vi "sub_prepare_HexPlot_command.vi"(10 "Dynamic data":T1, 11 "Input parameters":T2={"Measurement type"=enum."Debug", "Sensor type"=enum."HPK_8in_271ch", "Identifier"="test.txt", "Open after execution?"=FALSE, "Plot after execution?"=FALSE, "Display channel"=0, "Voltage Delay (s)"=0.5, "Switch Delay (s)"=0.01, "VISA resource name source"="", "VISA resource name DMM"="", "VISA resource name LCR"="", "Compliance  Level (A)"=10.0, "Voltage Limit (V)"=1000.0, "Data storage location"="", "Scan voltages"="", "Use source as DMM?"=FALSE, "LCR signal frequenzy (Hz)"=10.0, "DMM device"=enum."Keithley2001", "Sampling number"=1, "Use env. sensors on"=enum."Sensirion sht1x/7x", "Switchboard Handle"=0, "Use Switchboard"=FALSE, "LCR signal voltage (V)"=10000.0, "Repeat"=1, "Scan voltages IV"="", "Scan voltages CV"="", "Hex pad numbers?"=FALSE, "Set measurement type"=enum."Debug", "Custom pad scan"="", "IV voltage Delay (s)"=0.5, "CV voltage Delay (s)"=0.5, "Needle measurement?"=FALSE, "Comments"="test.txt", "LCR signal frequenzy (kHz)"=10.0, "Compliance  Level (uA)"=10.0, "Open Correction Array"=array2304x3[6912 elements], "Current set voltage"=0.0, "Last set voltage"=0.0, "Current channel"=0, "Last OpenCorrection index"=-1, "Total curr/vltg every x steps"=10, "Current channel iteration"=0, "No CV corrections"=FALSE, "Mapfile"="", "Corrfile"="", "IV voltage file"=path "", "CV voltage file"=path "", "IV Switch Delay (s)"=0.01, "CV Switch Delay (s)"=0.01, "Invert polarity"=FALSE, "Set debug dirs"=FALSE, "Is n on p"=FALSE, "Source interlock?"=TRUE, "Voltage file used?"=FALSE, "Pad mask"="", "Mask pad above (uA)"=1.0, "LCR device"=enum."LCR_E4980", "Source device"=enum."Source_2410", "HexPlot binary path"="", "PadReductionFactor"=1.0, "Temperature degC"="", "Fluence [neq]"="", "Annealing [min]"=""} {"CV Switch Delay (s)" format="%#_13g"; "IV Switch Delay (s)" format="%#_13g"; "Last set voltage" format="%#_13g"; "Current set voltage" format="%#_13g"; "CV voltage Delay (s)" format="%#_13g"; "IV voltage Delay (s)" format="%#_13g"; "Voltage Limit (V)" format="%#_13g"; "Voltage Delay (s)" format="%#_13g"; "Switch Delay (s)" format="%#_13g"}) -> (2 "Dynamic data out":T1)   [LabVIEW 2020]
doc: "Set HexPlot command for data display."
uses:
  input_params.ctl
  data_dynamic.ctl
panel:
  out "HexPlot analysis command":string
  out "HexPlot matrix command":string
  out "HexPlot command":string
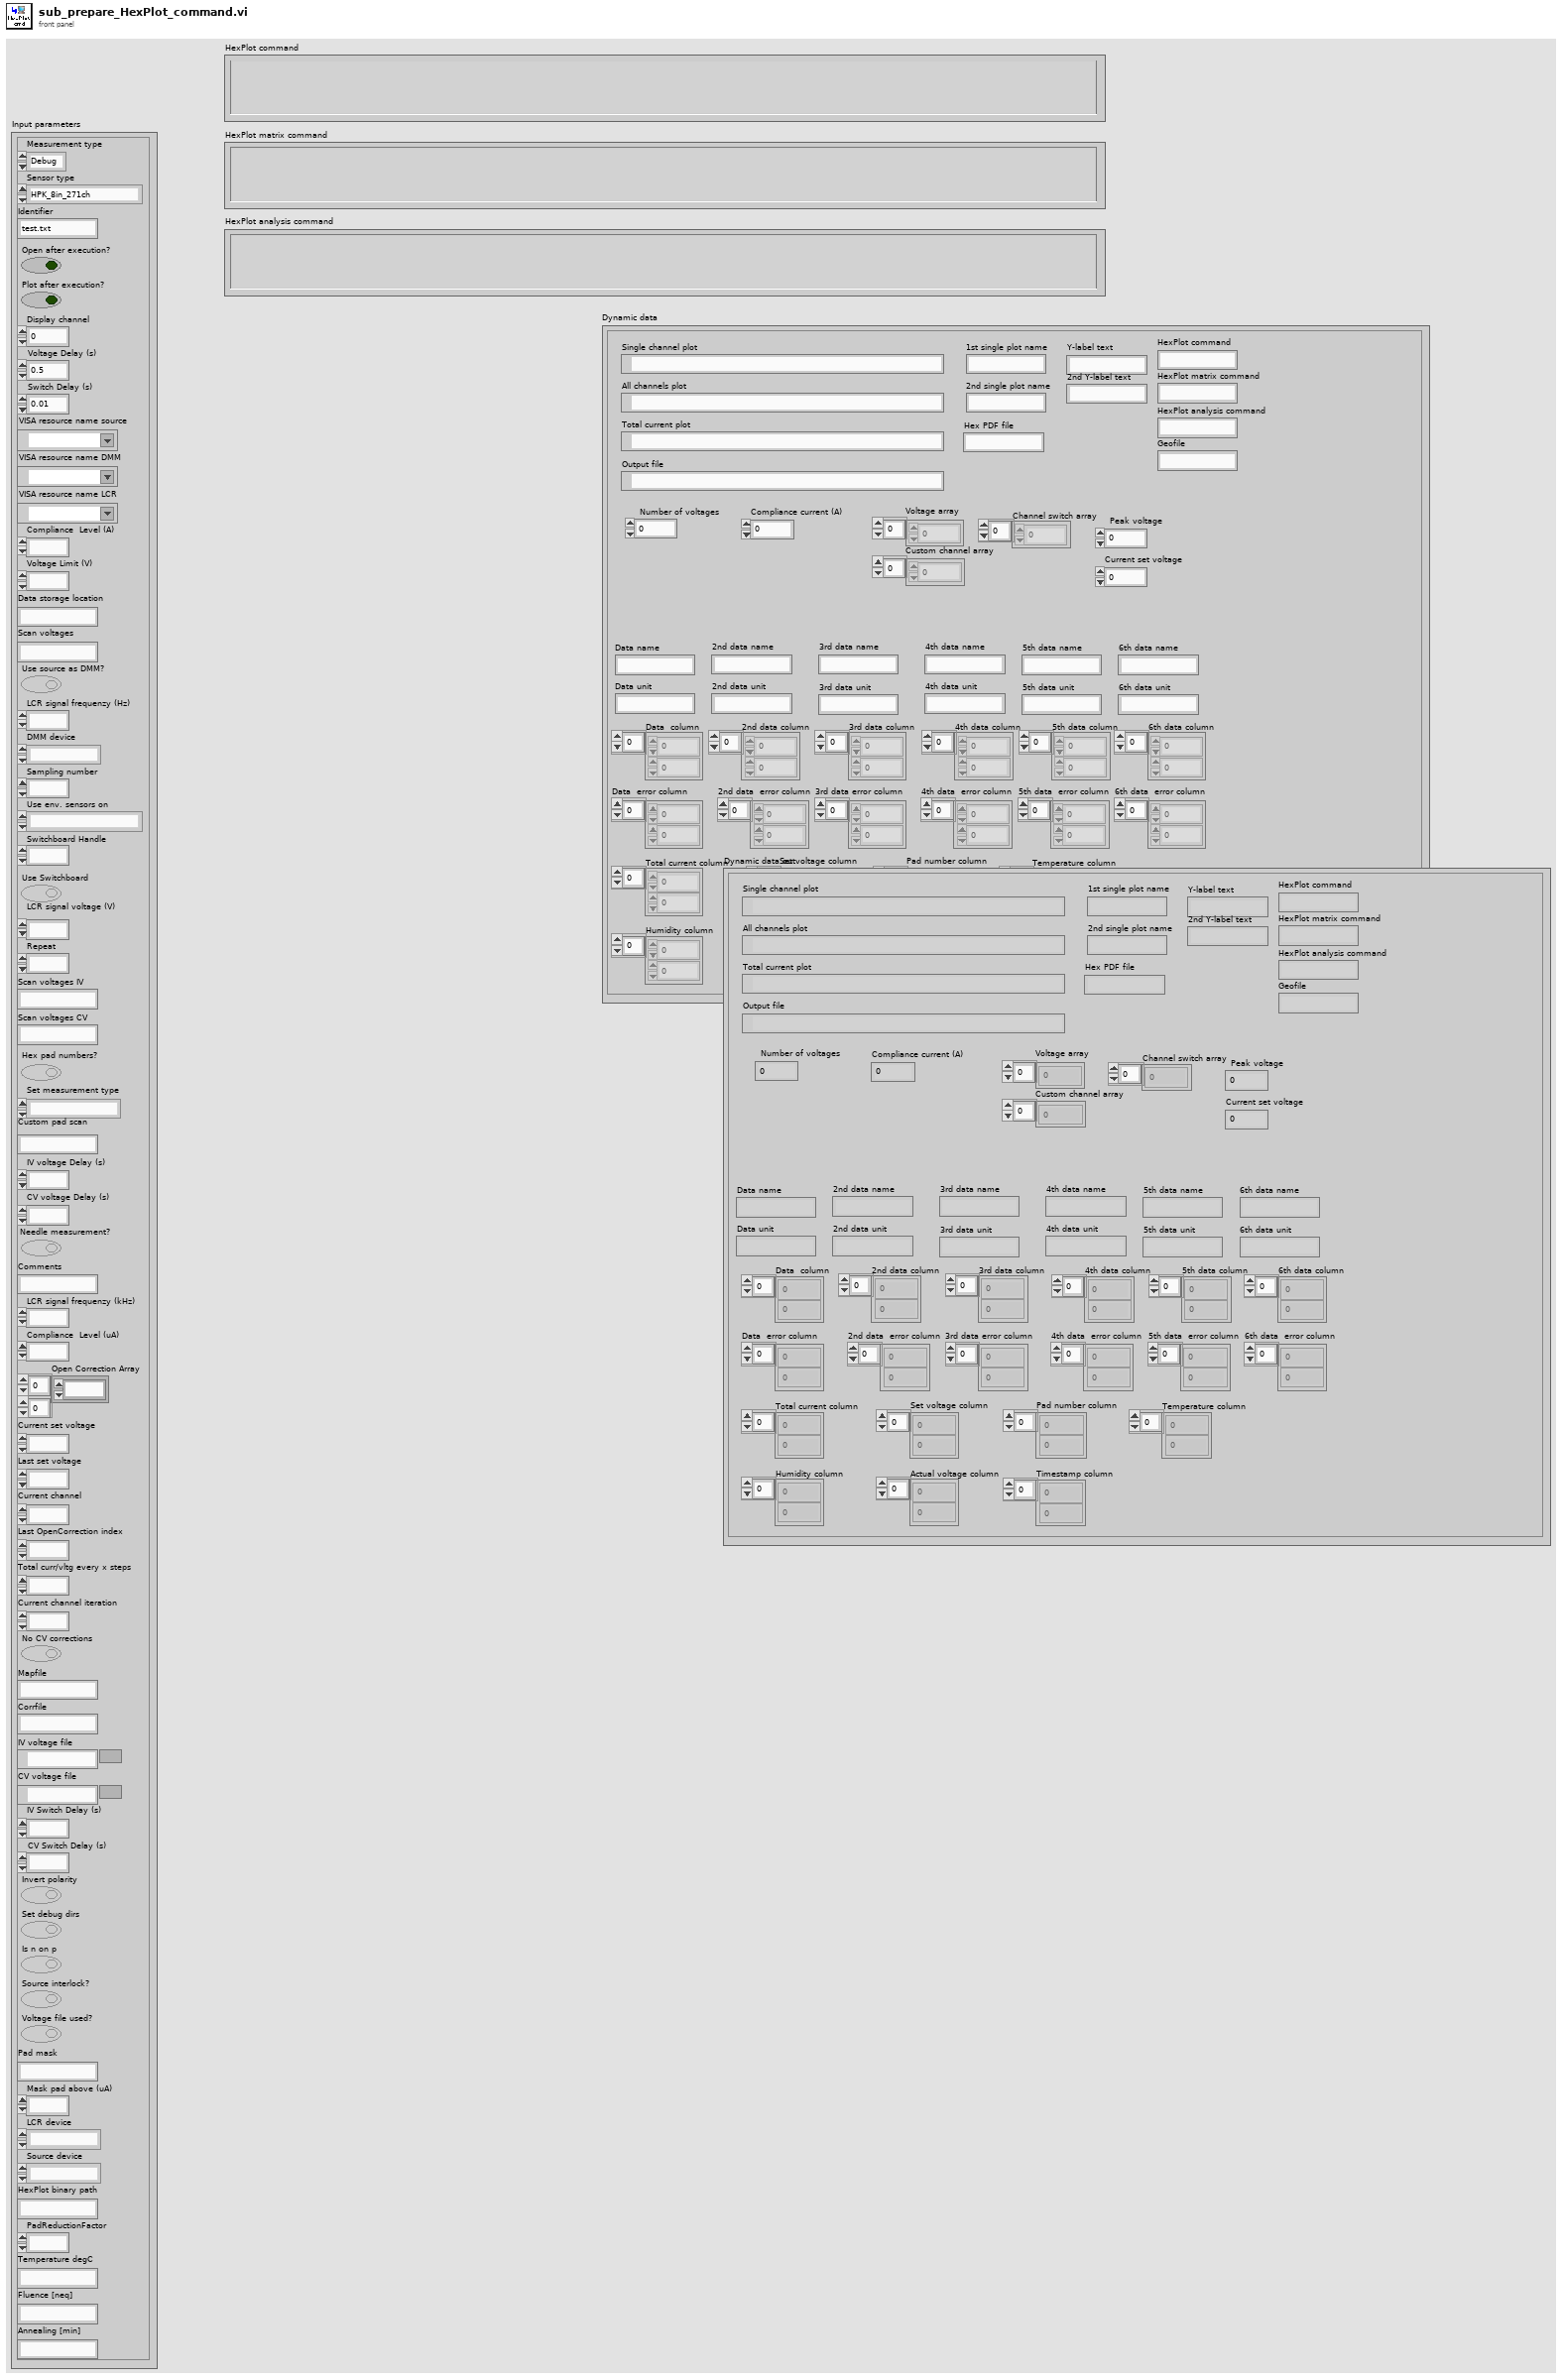
[diagram p1: front panel]
types:
  T1 = typedef "data_dynamic.ctl" = cluster{"Output file":path, "Y-label text":string, "Current set voltage":dbl, "Set voltage column":dbl[], "Pad number column":dbl[], "Data  column":dbl[], "Number of voltages":i32, "Compliance current (A)":dbl, "Geofile":string, "Peak voltage":dbl, "Hex PDF file":string, "Voltage array":dbl[], "Total current column":dbl[], "Timestamp column":dbl[], "Data name":string, "Data unit":string, "2nd data column":dbl[], "2nd data name":string, "2nd data unit":string, "3rd data column":dbl[], "4th data column":dbl[], "3rd data name":string, "3rd data unit":string, "4th data name":string, "4th data unit":string, "Actual voltage column":dbl[], "2nd Y-label text":string, "Single channel plot":path, "Temperature column":dbl[], "Humidity column":dbl[], "Channel switch array":i32[], "1st single plot name":string, "2nd single plot name":string, "All channels plot":path, "HexPlot command":string, "Custom channel array":i32[], "Data  error column":dbl[], "2nd data  error column":dbl[], "3rd data error column":dbl[], "4th data  error column":dbl[], "Total current plot":path, "5th data column":dbl[], "5th data  error column":dbl[], "6th data column":dbl[], "6th data  error column":dbl[], "5th data name":string, "5th data unit":string, "6th data name":string, "6th data unit":string, "HexPlot matrix command":string, "HexPlot analysis command":string}
  T2 = typedef "input_params.ctl" = cluster{"Measurement type":enum16{"IV", "CV", "Debug", "Test_contact"}, "Sensor type":enum16{"HPK_6in_135ch", "HPK_8in_271ch", "IFX_8in_256ch", "Diode", "HPK_6in_239ch", "Full_Matrix", "HPK_8in_271ch_full", "LumiCal", "HPK_8in_444ch", "HPK_8in_198ch_2019", "HPK_8in_MGW_LD_full", "HPK_8in_MGW_LD_a_type_top", "HPK_8in_MGW_LD_a_type_bottom", "HPK_8in_MGW_LD_b_type_left", "HPK_8in_MGW_LD_b_type_right", "HPK_8in_MGW_LD_c_type_left", "HPK_8in_MGW_LD_c_type_right", "HPK_8in_MGW_HD_full", "HPK_8in_MGW_HD_a_type_top", "HPK_8in_MGW_HD_a_type_bottom", "HPK_8in_MGW_HD_b_type_left", "HPK_8in_MGW_HD_b_type_right", "HPK_8in_MGW_HD_c_type_left", "HPK_8in_MGW_HD_c_type_right", "CALICE_6in_256ch"}, "Identifier":string, "Open after execution?":bool, "Plot after execution?":bool, "Display channel":i32, "Voltage Delay (s)":dbl, "Switch Delay (s)":dbl, "VISA resource name source":refnum<visa-resource-name>, "VISA resource name DMM":refnum<visa-resource-name>, "VISA resource name LCR":refnum<visa-resource-name>, "Compliance  Level (A)":dbl, "Voltage Limit (V)":dbl, "Data storage location":string, "Scan voltages":string, "Use source as DMM?":bool, "LCR signal frequenzy (Hz)":dbl, "DMM device":enum16{"Keithley2001", "Keithley2450", "Keithley2410", "Keithley6485", "Keithley6487", "Keithley6517"}, "Sampling number":i32, "Use env. sensors on":enum16{"Sensirion sht1x/7x", "Switch Matrix", "Probecard"}, "Switchboard Handle":u32, "Use Switchboard":bool, "LCR signal voltage (V)":dbl, "Repeat":i32, "Scan voltages IV":string, "Scan voltages CV":string, "Hex pad numbers?":bool, "Set measurement type":enum16{"IV", "CV", "Debug", "Test_contact", "IV+CV"}, "Custom pad scan":string, "IV voltage Delay (s)":dbl, "CV voltage Delay (s)":dbl, "Needle measurement?":bool, "Comments":string, "LCR signal frequenzy (kHz)":dbl, "Compliance  Level (uA)":dbl, "Open Correction Array":dbl[][], "Current set voltage":dbl, "Last set voltage":dbl, "Current channel":i32, "Last OpenCorrection index":i32, "Total curr/vltg every x steps":i32, "Current channel iteration":i32, "No CV corrections":bool, "Mapfile":string, "Corrfile":string, "IV voltage file":path, "CV voltage file":path, "IV Switch Delay (s)":dbl, "CV Switch Delay (s)":dbl, "Invert polarity":bool, "Set debug dirs":bool, "Is n on p":bool, "Source interlock?":bool, "Voltage file used?":bool, "Pad mask":string, "Mask pad above (uA)":dbl, "LCR device":enum16{"LCR_E4980", "AGILENT_4263X"}, "Source device":enum16{"Source_2410", "Source_6487", "Source_2470"}, "HexPlot binary path":string, "PadReductionFactor":dbl, "Temperature degC":string, "Fluence [neq]":string, "Annealing [min]":string}
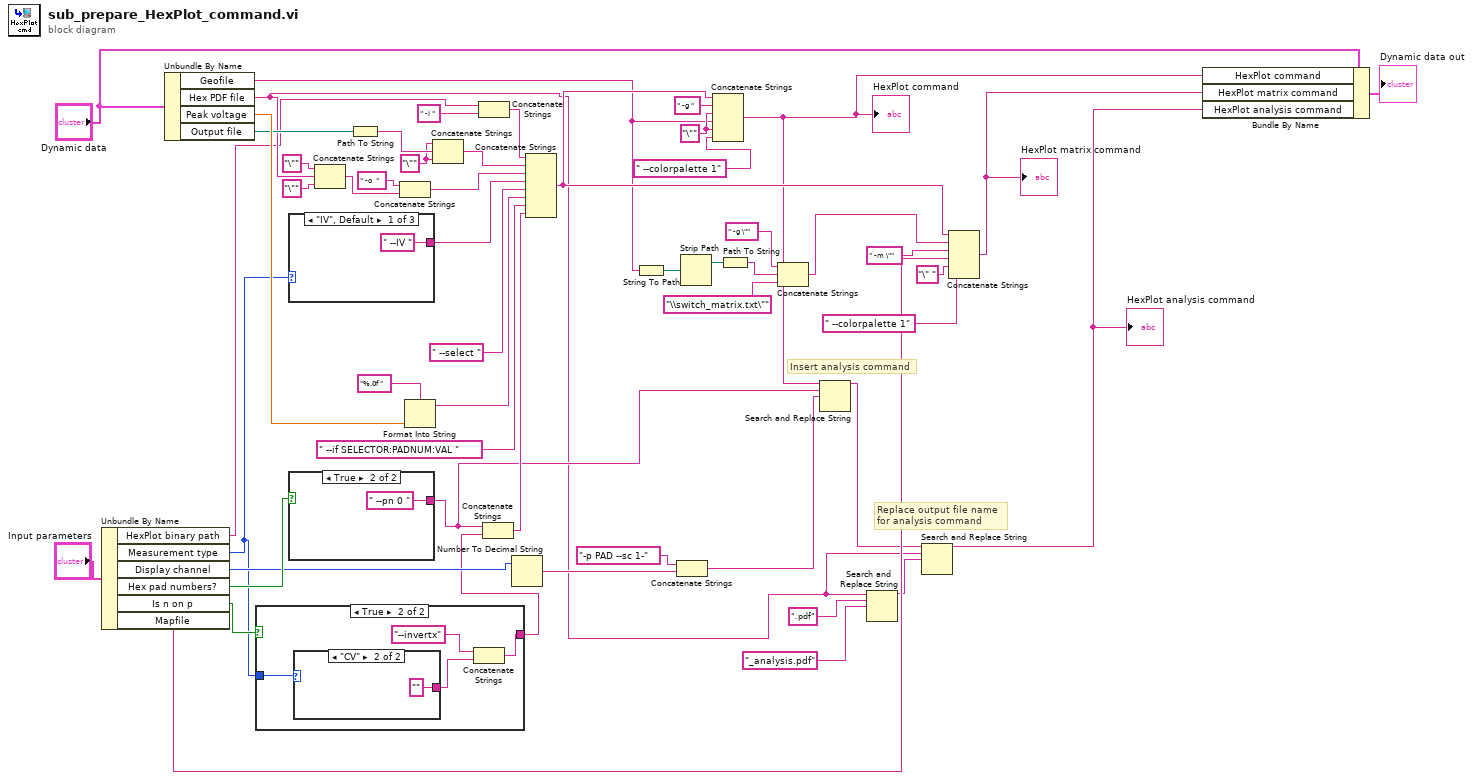
[diagram p0: block diagram]
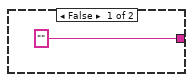
[diagram p2: hidden frame]
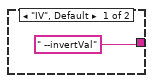
[diagram p3: hidden frame]
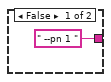
[diagram p4: hidden frame]
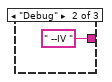
[diagram p5: hidden frame]
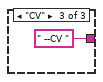
[diagram p6: hidden frame]
diagram:
  w33 = "\"" ("string")
  w32 = "\"" ("string")
  # "Replace output file name\nfor analysis command"
  # "Insert analysis command"
  n1 = Unbundle By Name("Input parameters") -> ("HexPlot binary path"=w3:string, "Measurement type"=w7:enum16{"IV", "CV", "Debug", "Test_contact"}, "Display channel"=w16:i32, "Hex pad numbers?"=w40:bool, "Is n on p"=w21:bool, "Mapfile"=w34:string)
  n2 = Unbundle By Name("Dynamic data") -> ("Geofile"=w29:string, "Hex PDF file"=w9:string, "Peak voltage"=w52:dbl, "Output file"=w41:path)
  n3 = case shown="True" w21 {
    tunnel: ["" ("string") w56] -> w6
    tunnel: w7 -> [_ w59]
    frame False {
    }
    frame True {
      n4 = case shown="\"CV\"" w59 {
        tunnel: [" --invertVal" ("string") "" ("string")] -> w58
        frame "IV", Default {
        }
        frame "CV" {
        }
      }
      n5 = Concatenate Strings("--invertx" ("string"), w58) -> (w56:string)
    }
  }
  n6 = case shown="\"IV\", Default" w7 {
    tunnel: [" --IV " ("string") " --IV " ("string") " --CV " ("string")] -> w54
    frame "IV", Default {
    }
    frame "Debug" {
    }
    frame "CV" {
    }
  }
  n7 = case shown="True" w40 {
    tunnel: [" --pn 1 " ("string") " --pn 0 " ("string")] -> w18
    frame False {
    }
    frame True {
    }
  }
  n8 = Concatenate Strings("\"" ("string"), w9, "\"" ("string")) -> (w43:string)
  n9 = Path To String(path=w41) -> (string=w42:string)
  n10 = Concatenate Strings(" -o  " ("string"), w43) -> (w47:string)
  n11 = Format Into String(format string="%.0f ", w52) -> (resulting string=w50:string)  [unwired: 2 in, 1 out]
  n12 = Concatenate Strings(w33, w42, w33) -> (w48:string)
  n13 = Concatenate Strings(w3, " -i " ("string")) -> (w5:string)
  n14 = Concatenate Strings(w18, w6) -> (w20:string)
  n15 = Number To Decimal String(number=w16) -> (decimal integer string=w15:string)  [unwired: 1 in]
  n16 = Concatenate Strings(w5, w48, w47, w54, " --select " ("string"), w50, " --if SELECTOR:PADNUM:VAL " ("string"), w20) -> (w30:string)
  n17 = String To Path(string=w29) -> (path=w28:path)
  n18 = Concatenate Strings("-p PAD --sc 1-" ("replace string (\"\")"), w15) -> (w14:string)
  n19 = Strip Path(path=w28) -> (stripped path=w27:path)  [unwired: 1 out]
  n20 = Concatenate Strings(w30, " -g " ("string"), w32, w29, w32, " --colorpalette 1") -> (w19:string)
  "HexPlot command" <- w19
  n21 = Path To String(path=w27) -> (string=w26:string)
  n22 = Concatenate Strings(" -g \"" ("string"), w26, "\\switch_matrix.txt\"" ("string")) -> (w24:string)
  n23 = Search and Replace String(input string=w19, search string=w18, replace string=w14) -> (result string=w13:string)  [unwired: 5 in, 3 out]
  n24 = Search and Replace String(input string=w9, search string=".pdf", replace string="_analysis.pdf" ("replace string (\"\")")) -> (result string=w10:string)  [unwired: 5 in, 3 out]
  n25 = Search and Replace String(input string=w13, search string=w9, replace string=w10) -> (result string=w8:string)  [unwired: 5 in, 3 out]
  "HexPlot analysis command" <- w8
  n26 = Concatenate Strings(w30, w24, " -m \"" ("string"), w34, "\" " ("string"), " --colorpalette 1") -> (w22:string)
  "HexPlot matrix command" <- w22
  n27 = Bundle By Name(cluster="Dynamic data", "HexPlot command"=w19, "HexPlot matrix command"=w22, "HexPlot analysis command"=w8) -> (→"Dynamic data out":T1)
